vi "WaitForReply.vi"(8 "ErrorIn":errorcluster, 9 "Name":string, 10 "ReplyQueue":refnum<queue>, 11 "Alive":refnum<queue>) -> (0 "ErrorOut":errorcluster, 2 "Reply":variant)   [LabVIEW 2021, in "YActor.lvclass"]
uses:
  YActor.lvclass
  CmdCtrl.ctl
  AsyncErrorHandling.ctl
  CallMode.ctl
  YActor.lvclass/YActor.ctl
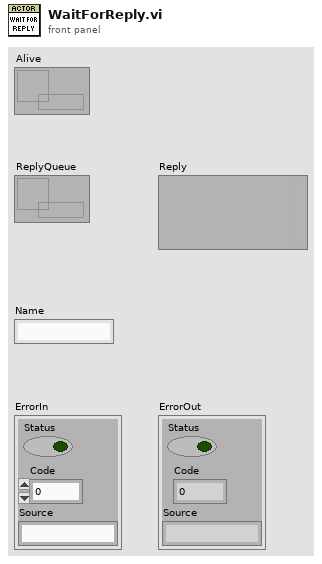
[diagram p1: front panel]
types:
  T1 = typedef "YActor.lvclass/CmdCtrl.ctl" = cluster{"CmdData":variant, "CommandVI":string, "ReplyQ":i64, "Error":errorcluster, "Msg#":u32, "Async Error Handling":T2, "CallMode":T3, "Source":string}
  T2 = typedef "YActor.lvclass/AsyncErrorHandling.ctl" = enum16{"Return after executing sync command", "Return before executing sync command", "Don't return error"}
  T3 = typedef "YActor.lvclass/CallMode.ctl" = enum16{"Standard", "Call&Collect"}
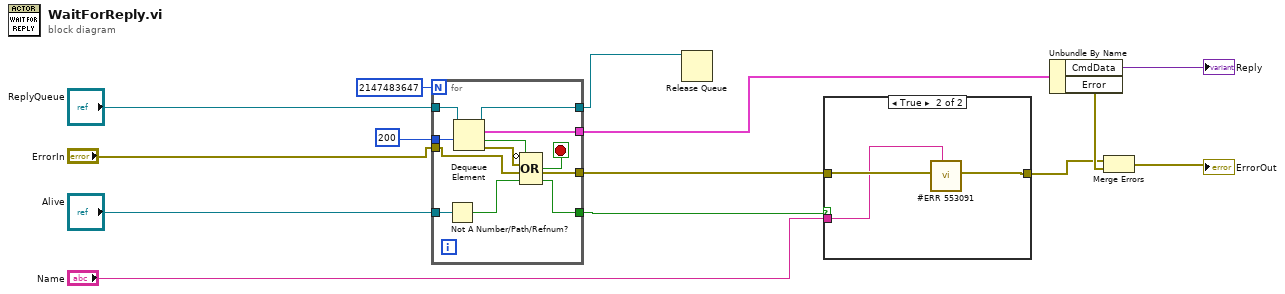
[diagram p0: block diagram]
diagram:
  n1 = for {
    N: 2147483647 -> [_]
    tunnel: [w22] -> w2
    tunnel: "Alive" -> [w16]
    tunnel: 200 ("Numeric") -> [w18]
    tunnel: "ErrorIn" -> [w23]
    tunnel: "ReplyQueue" -> [w21]
    tunnel: [w20] -> w7
    tunnel: [w23] -> w11
    tunnel: [w15] -> w3
    stop <- w19 stop-if-true
    n2 = Not A Number/Path/Refnum?(number/path/refnum=w16) -> (NaN/Path/Refnum?=w15:bool)
    n3 = Dequeue Element(queue=w21, timeout in ms (-1)=w18) -> (queue out=w20:refnum<queue>, element=w22:T1, timed out?=w17:bool, error out=w24:errorcluster)  [unwired: 1 in]
    n4 = Compound Arithmetic op=OR(invert w17, w24, w23, w15) -> (w19:bool)
  }
  n5 = Release Queue(queue=w7) -> ()  [unwired: 2 in, 3 out]
  n6 = case shown="True" w3 {
    tunnel: w11 -> [w25 w27]
    tunnel: "Name" -> [_ w26]
    tunnel: [w25 w28] -> w12
    frame False {
    }
    frame True {
      n7 = call "#ERR 553091"("Data"=w26, "error in (no error)"=w27) -> ("error out"=w28:errorcluster)  [unwired: 9 in]
    }
  }
  n8 = Unbundle By Name(w2) -> ("CmdData"=→"Reply":variant, "Error"=w13:errorcluster)
  n9 = Merge Errors(w12, w13) -> (→"ErrorOut":errorcluster)
